vi "Finished Collection Write File.vi"(0 "Output KPRO":path=path "c:/junk.dat", 1 "KPRO Culmulative \ntest report header 2":string[](array[string])=["Time(msecs)", "Uncorrected Depth", "Corrected Depth", "Drive_Rate", "Flow", "Feet_of Stainless", "Up Hole Pressure", "IK", "Corrected Pressure", "Atm Pressure", "Depth to water", "Height of box", "Res_Pressure", "Secs_since_1_JAN_1904", "Depth jumps more than 1_foot", "Down hole Pressure"], 3 "Replace File":bool, 5 "Feet of\nStainless to be\nUsed (Count) in":i32, 9 "Corrected Array in":dbl[][](array[numeric]), 12 "Cluster in":T1) -> (4 "Feet of\nStainless to be\nUsed (Count) out":i32, 6 "Depth to \nbe Used \n(Feet)":sgl, 10 "Corrected Array out":dbl[][](array[numeric]), 13 "Record IK Reason 2":bool, 14 "Array":u16[](array[numeric]))   [LabVIEW 2016]
uses:
  controls/Kpro hydraulic measurement cluster.ctl
  <vilib>/Utility/file.llb/Write Delimited Spreadsheet (string).vi
  <vilib>/Utility/file.llb/Write Delimited Spreadsheet (DBL).vi
panel:
  in  "Select Entry \nfor IK Log":u16(ring) items=["IK Increase", "IK stayed the Same", "IK decreased"]
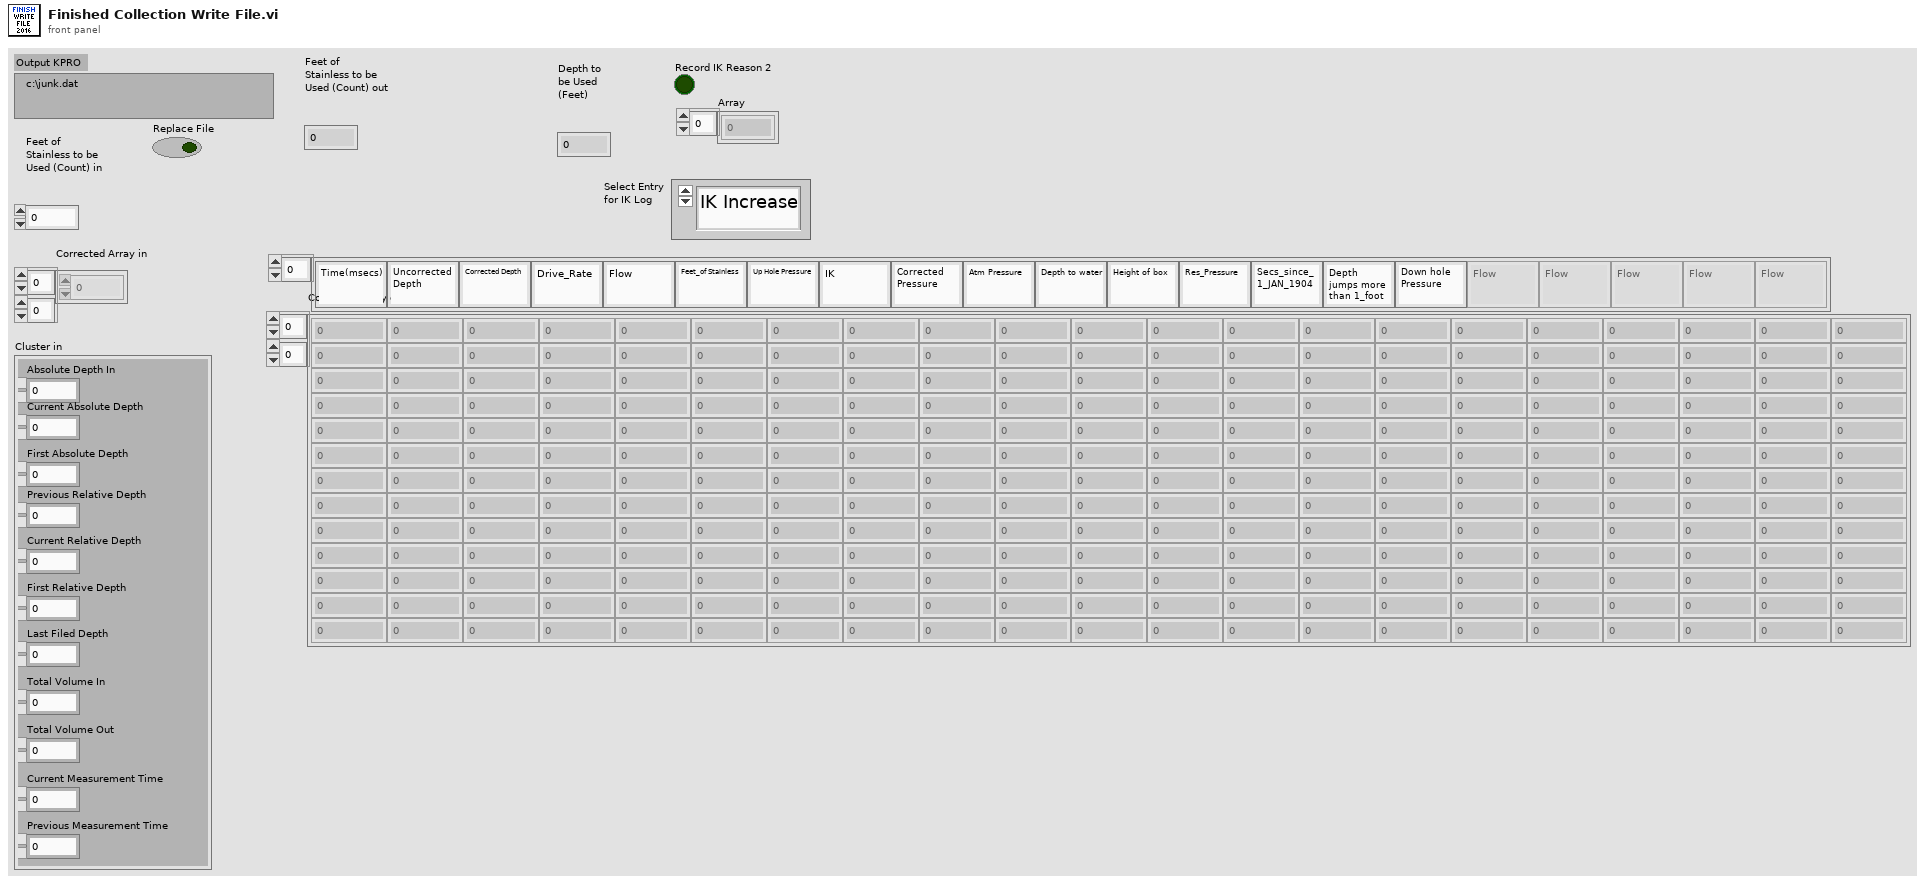
[diagram p1: front panel]
types:
  T1 = typedef "Kpro hydraulic measurement cluster.ctl" = cluster{"Absolute Depth In":dbl, "Current Absolute Depth":dbl, "First Absolute Depth":dbl, "Previous Relative Depth":dbl, "Current Relative Depth":dbl, "First Relative Depth":dbl, "Last Filed Depth":dbl, "Total Volume In":dbl, "Total Volume Out":dbl, "Current Measurement Time":dbl, "Previous Measurement Time":dbl}
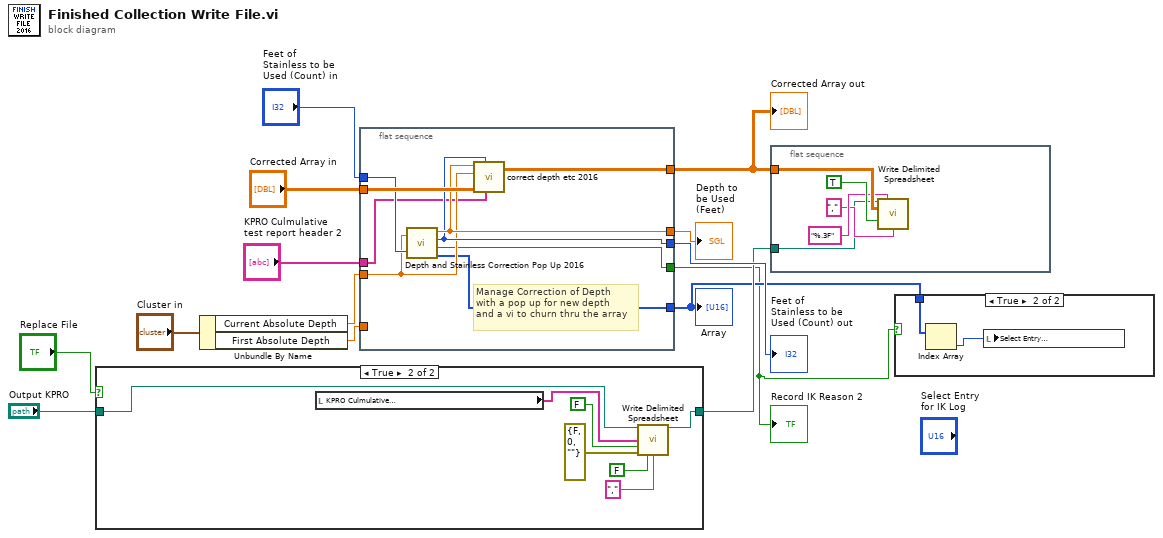
[diagram p0: block diagram]
diagram:
  n1 = case shown="True" "Replace File" {
    tunnel: "Output KPRO" -> [w15 w22]
    tunnel: [w15 w18] -> w5
    frame False {
    }
    frame True {
      n2 = local read "KPRO Culmulative \ntest report header 2"() -> (w16:string[])
      n3 = call-poly <vilib>:"Write Delimited Spreadsheet.vi"("file path (dialog if empty)"=w22, "1D data"=w16, "append to file? (new file:F)"=FALSE, "error in (no error)"=errorcluster {"status"=FALSE, "code"=0, "source"=""} ("error constant"), "transpose? (no:F)"=FALSE, "delimiter (\\t)"="," ("delimiter (\\t)")) -> ("new file path (Not A Path if cancelled)"=w18:path)  [unwired: 8 in, 1 out]
    }
  }
  n4 = Unbundle By Name("Cluster in") -> ("Current Absolute Depth"=w13:dbl, "First Absolute Depth"=w14:dbl)
  n5 = flat-sequence {
    tunnel: "Corrected Array in" -> [w31]
    tunnel: [w30] -> w8
    tunnel: w14 -> [_]
    tunnel: [w29] -> w9
    tunnel: "Feet of\nStainless to be\nUsed (Count) in" -> [w28]
    tunnel: [w27] -> w11
    tunnel: w13 -> [w26]
    tunnel: [w25] -> w1
    tunnel: [w24] -> w2
    tunnel: "KPRO Culmulative \ntest report header 2" -> [w23]
    frame #0 {
      # "Manage Correction of Depth\nwith a pop up for new depth\nand a vi to churn thru the array"
      n6 = call "Depth and Stainless Correction Pop Up 2016.vi"("Input \nCorrected \nDepth (Feet)"=w26, "New Number\n of Stainless\n(Count)"=w28) -> ("Depth to \nbe Used \n(Feet)"=w30:sgl, "Feet of\nStainless to be\nUsed (Count)"=w27:i32, "Record IK Reason 2"=w25:bool, "Array"=w24:u16[])
      n7 = call "correct depth etc 2016.vi"("KPRO Culmulative \ntest report header 2"=w23, "New Stainless Feet"=w27, "Cumulative_data_in"=w31, "Incorrect Depth"=w26, "Correct Depth"=w30) -> ("Cumulative_data_out"=w29:dbl[][])  [unwired: 2 in]
    }
  }
  n8 = flat-sequence {
    tunnel: w9 -> [w35]
    tunnel: w5 -> [w32]
    frame #0 {
      n9 = call-poly <vilib>:"Write Delimited Spreadsheet.vi"("file path (dialog if empty)"=w32, "format (%.3f)"="%.3F", "2D data"=w35, "append to file? (new file:F)"=TRUE, "delimiter (\\t)"="," ("delimiter (\\t)")) -> ()  [unwired: 9 in, 2 out]
    }
  }
  n10 = case shown="True" w1 {
    tunnel: w2 -> [_ w38]
    frame False {
    }
    frame True {
      n11 = Index Array(array=w38) -> (element=w37:u16)  [unwired: 1 in]
      n12 = local write "Select Entry \nfor IK Log"(w37) -> ()
    }
  }
  "Feet of\nStainless to be\nUsed (Count) out" <- w11
  "Corrected Array out" <- w9
  "Depth to \nbe Used \n(Feet)" <- w8
  "Record IK Reason 2" <- w1
  "Array" <- w2
